vi "MethodSCRIPTExample.vi"() -> ()   [LabVIEW 2025]
uses:
  PalmSens/PalmSens.lvclass
  E:/PSCode/PalmSens_SDK/labview/PalmSens/Libraries/PalmSens.Core.Simplified.LabVIEW.dll
  PalmSens/Libraries/PalmSens.Core.Simplified.LabVIEW.dll
  PalmSens/MeasurementResults.ctl
  PalmSens/LiveCurveResult.ctl
panel:
  out "Curves":T1
  out "MethodSCRIPT":refnum<k24>
  out "Array":string[](array[string])
  out "Is Measuring":bool
  in  "PalmSens.lvclass":refnum<class "PalmSens.lvclass">
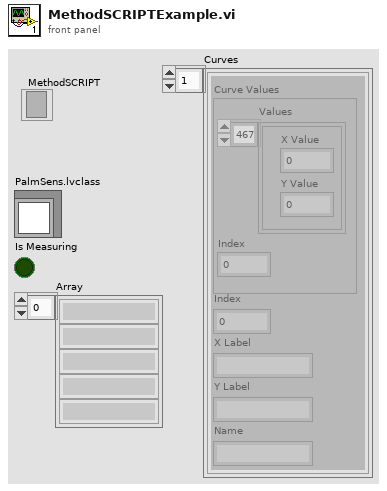
[diagram p1: front panel]
types:
  T1 = typedef "MeasurementResults.ctl" = T2[]
  T2 = typedef "LiveCurveResult.ctl" = cluster{"X Label":string, "Y Label":string, "Name":string, "Index":i16, "Curve Values":cluster{"Values":cluster{"X Value":dbl, "Y Value":dbl}[], "Index":i16}}
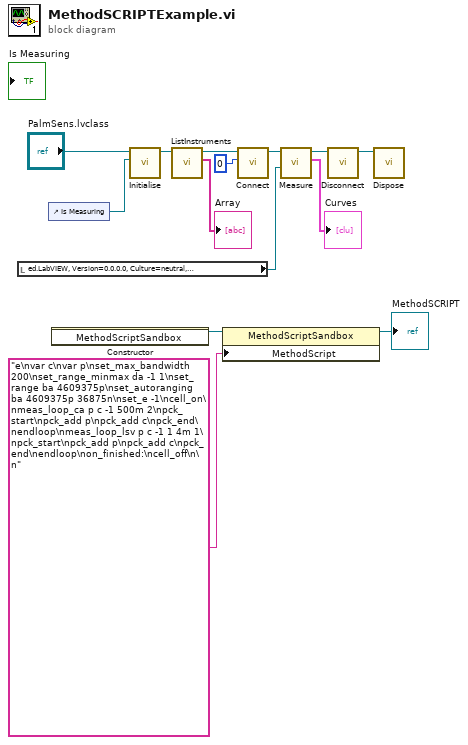
[diagram p0: block diagram]
diagram:
  n1 = local read "MethodSCRIPT"() -> (w1:refnum<k24>)
  n2 = control-ref of="Is Measuring"() -> (w13:refnum<vi>)
  n3 = constructor class="MethodScriptSandbox"() -> (reference out=w7:refnum<k24>)  [unwired: 3 in, 2 out]
  n4 = call-dynamic "Initialise.vi"("Is Measuring Refnum"=w13, "PalmSens in"="PalmSens.lvclass") -> ("PalmSens out"=w12:refnum<class "PalmSens.lvclass">)  [unwired: 8 in, 1 out]
  n5 = call-dynamic "ListInstruments.vi"("PalmSens in"=w12) -> ("Array"=→"Array":string[], "PalmSens out"=w10:refnum<class "PalmSens.lvclass">)  [unwired: 8 in, 1 out]
  n6 = property class="MethodScriptSandbox"(reference=w7, "MethodScript"="e\nvar c\nvar p\nset_max_bandwidth 200\nset_range_minmax da -1 1\nset_range ba 4609375p\nset_autoranging ba 4609375p 36875n\nset_e -1\ncell_on\nmeas_loop_ca p c -1 500m 2\npck_start\npck_add p\npck_add c\npck_end\nendloop\nmeas_loop_lsv p c -1 1 4m 1\npck_start\npck_add p\npck_add c\npck_end\nendloop\non_finished:\ncell_off\n\n") -> (reference out=→"MethodSCRIPT":refnum<k24>)  [unwired: 1 in, 1 out]
  n7 = call-dynamic "Connect.vi"("Instrument Index"=0, "PalmSens in"=w10) -> ("PalmSens out"=w4:refnum<class "PalmSens.lvclass">)  [unwired: 8 in, 1 out]
  n8 = call-dynamic "Measure.vi"("Method .NET Refnum"=w1, "PalmSens in"=w4) -> ("Curves"=→"Curves":T1, "PalmSens out"=w3:refnum<class "PalmSens.lvclass">)  [unwired: 2 in, 2 out]
  n9 = call-dynamic "Disconnect.vi"("PalmSens in"=w3) -> ("PalmSens out"=w8:refnum<class "PalmSens.lvclass">)  [unwired: 9 in, 1 out]
  n10 = call-dynamic "Dispose.vi"("PalmSens in"=w8) -> ()  [unwired: 9 in, 2 out]
